vi "loadHist.vi"(11 "folder":string="QAMT01\\CRH3605") -> (0 "f":bool)   [LabVIEW 2012]
panel:
  out "Output 2":string
  out "OK":bool
  out "Output":string
  out "error out":errorcluster
  in  "error in (no error)":errorcluster
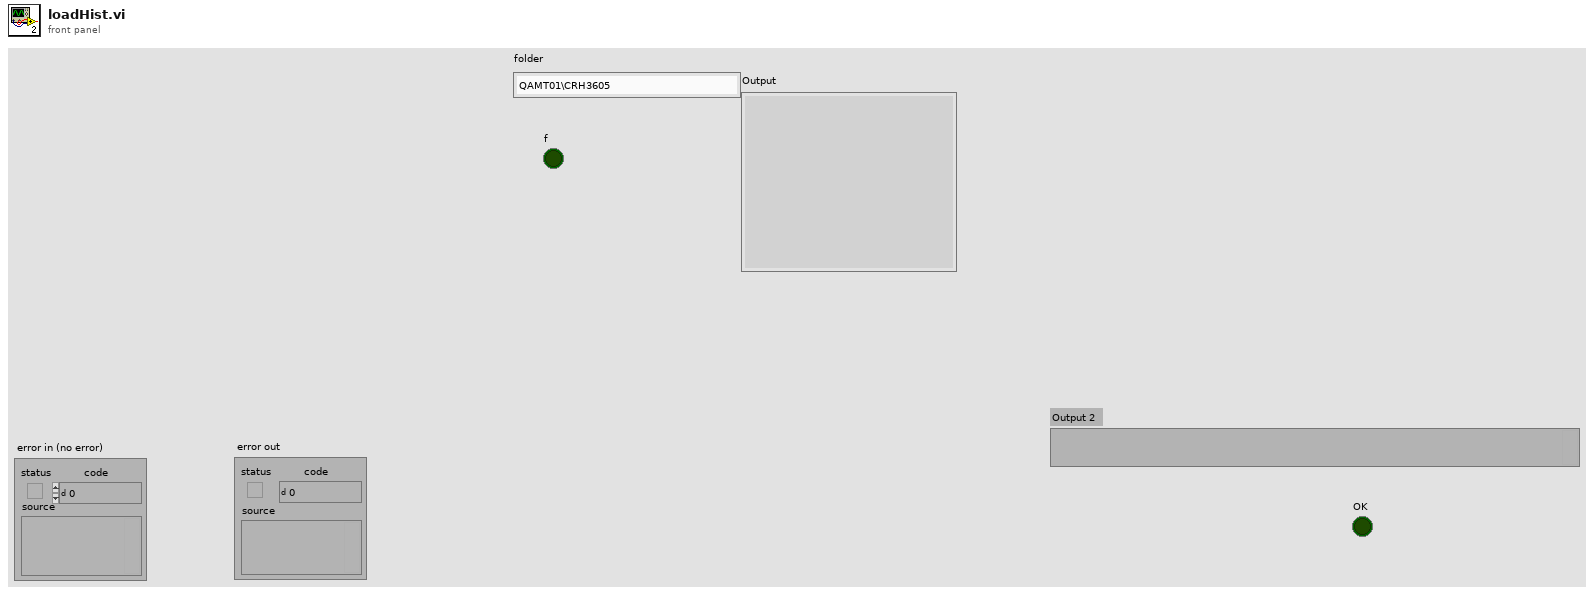
[diagram p1: front panel]
types:
  T1 = enum16{"open", "replace", "create", "open or create", "replace or create", "replace or create with confirmation"}
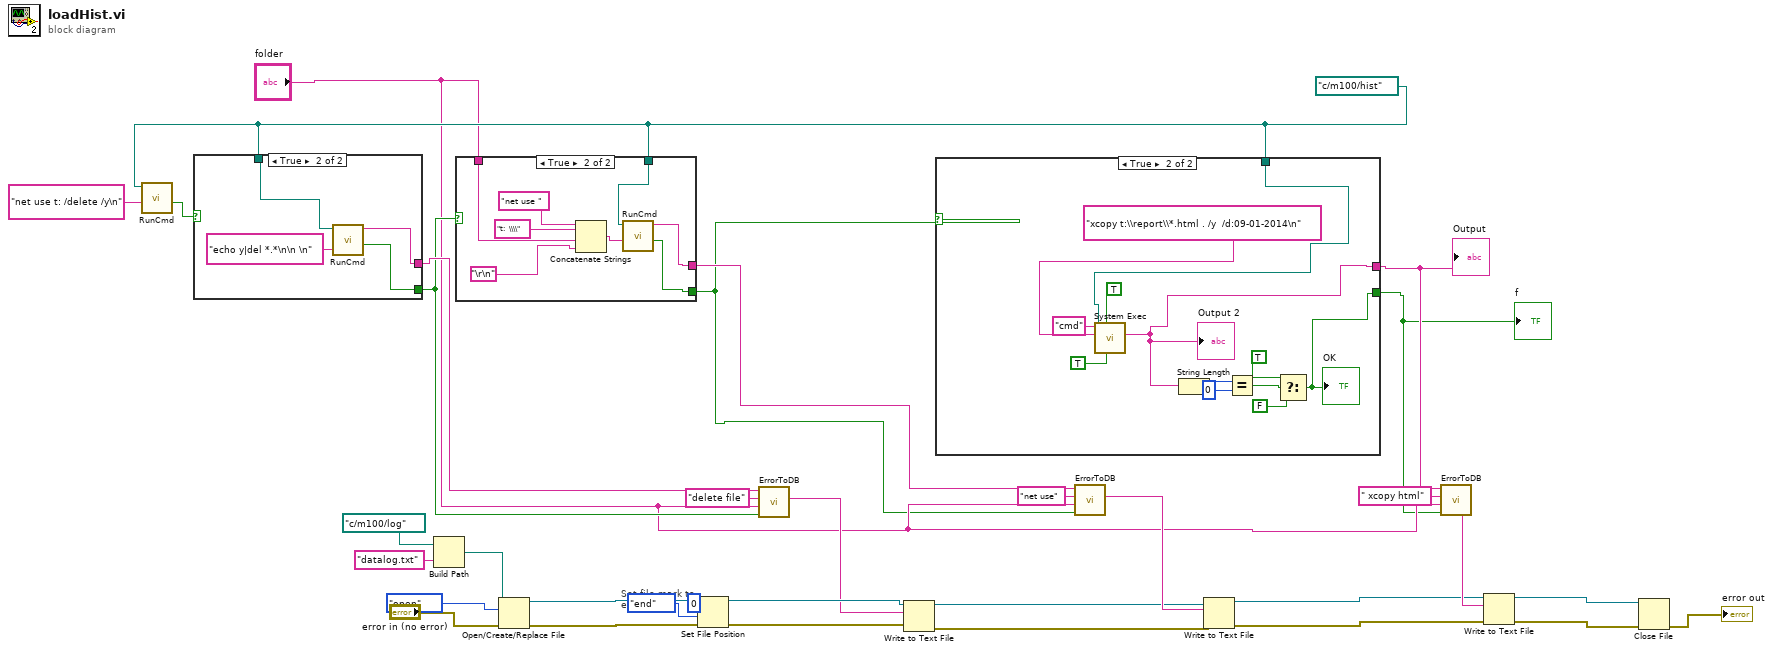
[diagram p0: block diagram]
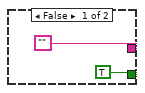
[diagram p2: hidden frame]
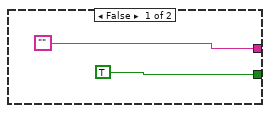
[diagram p3: hidden frame]
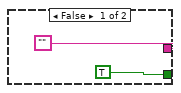
[diagram p4: hidden frame]
diagram:
  w19 = path "c:/m100/hist" ("base path")
  # "Set file mark to\nend of file"
  n1 = call "RunCmd.vi"("Cmd String"="net use t: /delete /y\n" ("string"), "working directory"=w19) -> ("OK"=w18:bool)  [unwired: 8 in, 1 out]
  n2 = case shown="True" w18 {
    tunnel: [TRUE w38] -> w12
    tunnel: ["" w37] -> w13
    tunnel: w19 -> [_ w40]
    frame False {
    }
    frame True {
      n3 = call "RunCmd.vi"("Cmd String"="echo y|del *.*\n\n \n" ("standard input"), "working directory"=w40) -> ("OK"=w38:bool, "Output"=w37:string)  [unwired: 8 in]
    }
  }
  n4 = Build Path(base path=path "c:/m100/log" ("path"), name or relative path="datalog.txt") -> (appended path=w25:path)
  n5 = case shown="True" w12 {
    tunnel: [TRUE w43] -> w6
    tunnel: ["" w44] -> w22
    tunnel: "folder" -> [_ w46]
    tunnel: w19 -> [_ w45]
    frame False {
    }
    frame True {
      n6 = Concatenate Strings("net use " ("string"), "t:  \\\\" ("string"), w46, "\r\n") -> (w50:string)
      n7 = call "RunCmd.vi"("Cmd String"=w50, "working directory"=w45) -> ("OK"=w43:bool, "Output"=w44:string)  [unwired: 8 in]
    }
  }
  n8 = Open/Create/Replace File(file path (use dialog)=w25, error in="error in (no error)", operation (0:open)=T1."open") -> (refnum out=w30:refnum<file>, error out=w29:errorcluster)  [unwired: 3 in, 1 out]
  n9 = Set File Position(offset (in bytes) (0)=i64 0, refnum=w30, from (0:start)=enum16{"start", "end", "current"}."end", error in=w29) -> (refnum out=w17:refnum<file>, error out=w16:errorcluster)
  n10 = call "ErrorToDB.vi"("Error"=w12, "Folder"="folder", "Command"="delete file", "Error Message"=w13) -> ("LogData"=w11:string)  [unwired: 7 in]
  n11 = Write to Text File(file (use dialog)=w17, text=w11, error in=w16) -> (refnum out=w15:refnum<file>, error out=w14:errorcluster)  [unwired: 1 in, 1 out]
  n12 = case shown="True" w6 {
    tunnel: [TRUE w55] -> w1
    tunnel: ["" w53] -> w21
    tunnel: w19 -> [_ w56]
    frame False {
    }
    frame True {
      n13 = call <vilib>:"System Exec.vi"("run minimized? (F)"=TRUE, "wait until completion? (T)"=TRUE, "working directory"=w56, "standard input"="xcopy t:\\report\\*.html . /y  /d:09-01-2014\n" ("string"), "command line"="cmd") -> ("standard error"=w53:string)  [unwired: 1 in, 5 out]
      "Output 2" <- w53
      n14 = String Length(string=w53) -> (length=w60:i32)
      n15 = Equal?(x=w60, y=0) -> (x = y?=w62:bool)
      n16 = Select(t=TRUE, s=w62, f=FALSE) -> (s? t:f=w55:bool)
      "OK" <- w55
    }
  }
  "f" <- w1
  "Output" <- w21
  n17 = call "ErrorToDB.vi"("Error"=w6, "Folder"="folder", "Command"="net use", "Error Message"=w22) -> ("LogData"=w24:string)  [unwired: 7 in]
  n18 = Write to Text File(file (use dialog)=w15, text=w24, error in=w14) -> (refnum out=w5:refnum<file>, error out=w4:errorcluster)  [unwired: 1 in, 1 out]
  n19 = call "ErrorToDB.vi"("Error"=w1, "Folder"="folder", "Command"=" xcopy html", "Error Message"=w21) -> ("LogData"=w20:string)  [unwired: 7 in]
  n20 = Write to Text File(file (use dialog)=w5, text=w20, error in=w4) -> (refnum out=w3:refnum<file>, error out=w2:errorcluster)  [unwired: 1 in, 1 out]
  n21 = Close File(refnum=w3, error in=w2) -> (error out=→"error out":errorcluster)  [unwired: 1 out]
